vi "MoAgSy_AgentBase_MSGhandler.vi"(0 "HGF_Agent in":refnum<class "MoAgSy_AgentBase.lvclass">, 2 "MoAgSy_Message":refnum<class "MoAgSy_Message.lvclass">, 5 "error in (no error)":errorcluster) -> (14 "HGF_Agent out":refnum<class "MoAgSy_AgentBase.lvclass">, 19 "error out":errorcluster)   [LabVIEW 2009, in "MoAgSy_Base.lvlib" / "MoAgSy_AgentBase.lvclass"]
uses:
  MoAgSy_AgentBase.lvclass
  MoAgSy_Message/MoAgSy_Message.lvclass
  MoAgSy_AgentBase.lvclass/MoAgSy_AgentBase.ctl
  MoAgSy_GPG/MoAgSy_GPG.lvclass
  HGF_BaseClasses/HGF_Factory/HGF_Factory.lvclass
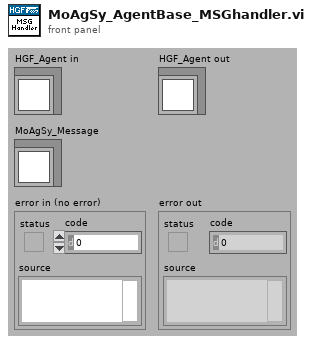
[diagram p1: front panel]
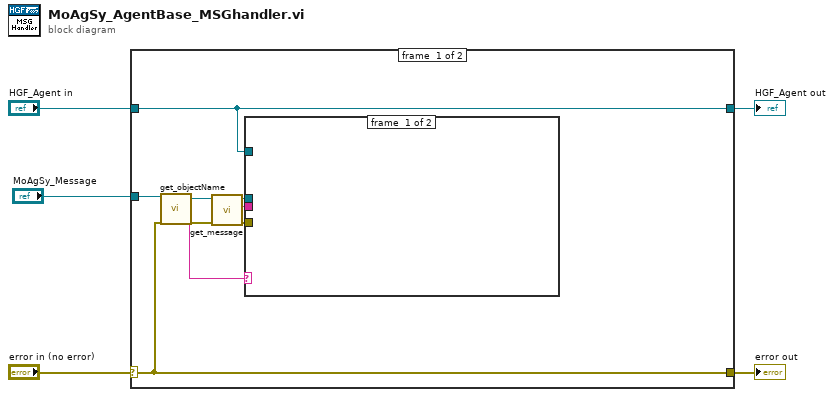
[diagram p0: block diagram]
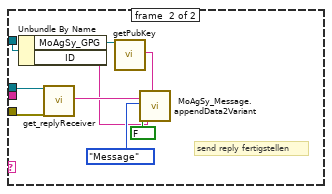
[diagram p2: hidden frame]
diagram:
  n1 = case shown="No Error" "error in (no error)" {
    selector: "error in (no error)" -> [w6 w25]
    tunnel: [w6 w25] -> w4
    tunnel: [w7 w24] -> w2
    tunnel: "HGF_Agent in" -> [w7 w24]
    tunnel: "MoAgSy_Message" -> [w14 _]
    frame #0 {
      n2 = call "get_objectName.vi"("HGF_Factory"=w14, "error in (no error)"=w6) -> ("dup HGF_Factory"=w13:refnum<class "MoAgSy_Message.lvclass">, "objectName"=w12:string, "error out"=w9:errorcluster)  [unwired: 15 in]
      n3 = call "get_message.vi"("error in (no error)"=w9, "MoAgSy_Message.lvclass in"=w13) -> ("error out"=w8:errorcluster, "Message"=w10:string, "MoAgSy_Message.lvclass out"=w11:refnum<class "MoAgSy_Message.lvclass">)  [unwired: 7 in]
      n4 = case shown="\"Pub Key request\"" w12 {
        tunnel: w11 -> [_ w23]
        tunnel: w10 -> [_ _]
        tunnel: w8 -> [_ w22]
        tunnel: w7 -> [_ w21]
        frame #0 {
        }
        frame #1 {
          # "send reply fertigstellen"
          n5 = Unbundle By Name(w21) -> ("MoAgSy_GPG"=w20:refnum<class "MoAgSy_GPG.lvclass">, "ID"=w15:string)
          n6 = call "get_replyReceiver.vi"("MoAgSy_Message"=w23, "error in (no error)"=w22) -> ("reply to"=w18:string)  [unwired: 12 in, 5 out]
          n7 = call-dynamic "getPubKey.vi"("HGF_GPG.lvclass in"=w20) -> ("public Key"=w19:string)  [unwired: 16 in, 2 out]
          n8 = call "MoAgSy_Message.appendData2Variant.vi"("addressee"=w18, "type"=enum16{"mobile Agent", "Visitor", "Message"}."Message", "request reply"=FALSE, "sender"=w15, "message"=w19) -> ()  [unwired: 13 in, 2 out]
        }
      }
    }
    frame #1 {
    }
  }
  "error out" <- w4
  "HGF_Agent out" <- w2
